vi "writeToXML.vi"(8 "error in (no error)":errorcluster, 10 "ClassLabel":string, 11 "ClearOffset in":refnum<class "ClearOffset.lvclass">) -> (0 "error out":errorcluster, 2 "XML out":string, 3 "ClearOffset out":refnum<class "ClearOffset.lvclass">)   [LabVIEW 2014, in "TCSDataDefinitions.lvlib" / "TCSCommand.lvlib" / "OffsetCommands.lvlib" / "ClearOffset.lvclass"]
uses:
  ClearOffset.lvclass
  ClearOffset.lvclass/ClearOffset.ctl
  TargetOffsetCommands/TargetOffsetCommands.lvclass
  <userlib>/Common/XML/XMLGenerator/XMLGenerator.lvclass
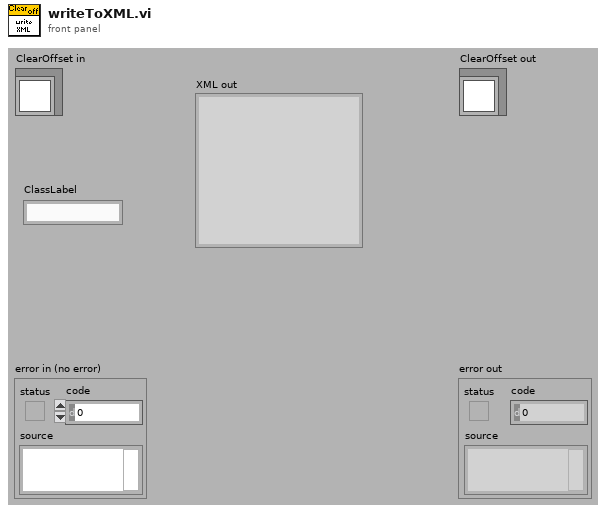
[diagram p1: front panel]
types:
  T1 = typedef "TCSDataDefinitions.lvlib/TCSCommand.lvlib/OffsetCommands.lvlib/Num2Types.ctl" = enum16{"User", "Handset", "Both"}
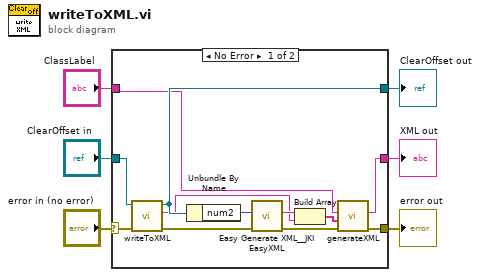
[diagram p0: block diagram]
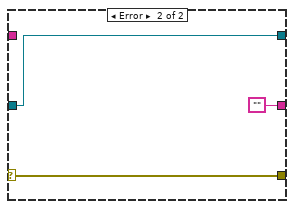
[diagram p2: hidden frame]
diagram:
  n1 = case shown="No Error" "error in (no error)" {
    selector: "error in (no error)" -> [w17 w21]
    tunnel: [w10 w21] -> w5
    tunnel: [w16 w20] -> w3
    tunnel: "ClearOffset in" -> [w18 w20]
    tunnel: "ClassLabel" -> [w8 _]
    tunnel: [w9 ""] -> w1
    frame No Error {
      n2 = call-parent "writeToXML.vi"("error in (no error)"=w17, "TargetOffsetCommands in"=w18) -> ("error out"=w14:errorcluster, "XML out"=w7:string, "TargetOffsetCommands out"=w16:refnum<class "ClearOffset.lvclass">)  [unwired: 7 in]
      n3 = Unbundle By Name(w16) -> ("num2"=w15:T1)
      n4 = call <vilib>:"Easy Generate XML__JKI EasyXML.vi"("error in (no error)"=w14, "LabVIEW Data"=w15) -> ("error out"=w11:errorcluster, "XML String"=w12:string)  [unwired: 8 in]
      n5 = Build Array(w12, w7) -> (w13:string[])
      n6 = call <userlib>:"generateXML.vi"("error in"=w11, "childrenXML"=w13, "elementName"=w8) -> ("error out"=w10:errorcluster, "XML out"=w9:string)  [unwired: 6 in, 1 out]
    }
    frame Error {
    }
  }
  "error out" <- w5
  "ClearOffset out" <- w3
  "XML out" <- w1
